vi "Temp Array Gen.2.vi"() -> ()   [LabVIEW 2014]
doc: "Temp Array Gen\n\nCreates an array of temperature given the starting, step, end temperature. This should return an array and the number of temperatures. Takes in consideration inverted limits and steps of zero.\n\nBeverly Abadines\nPHY 350 \nBAP3B"
uses:
  typedefs/temp control params.ctl
panel:
  out "error out":errorcluster
  in  "error in (no error)":errorcluster
  in  "Temperature Control Parameters":T1 {"End Temp" format="%.2f"; "Temp Step" format="%.2f"; "Start Temp" format="%.2f"}
  out "N Temps":i32=6
  out "Temp Array":dbl[](array[numeric])
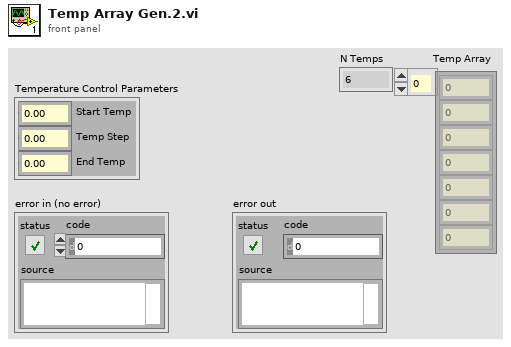
[diagram p1: front panel]
types:
  T1 = typedef "temp control params.ctl" = cluster{"Start Temp":dbl, "Temp Step":dbl, "End Temp":dbl}
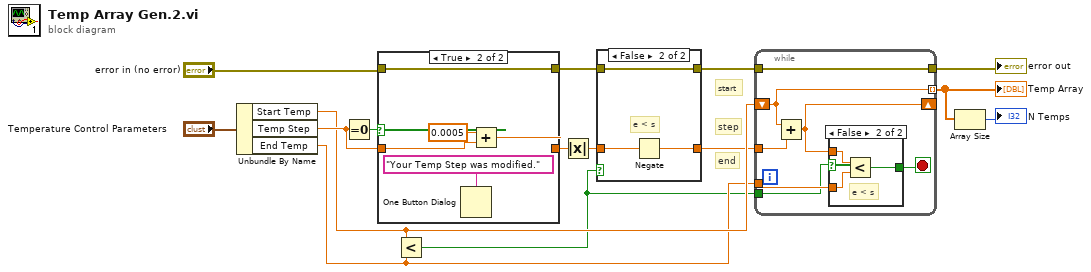
[diagram p0: block diagram]
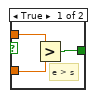
[diagram p4: hidden frame]
diagram:
  # "end"
  # "step"
  # "start"
  n1 = Unbundle By Name("Temperature Control Parameters") -> ("Start Temp"=w8:dbl, "Temp Step"=w11:dbl, "End Temp"=w7:dbl)
  n2 = Equal To 0?(x=w11) -> (x = 0?=w12:bool)
  n3 = case shown="True" w12 {
    tunnel: w11 -> [w17 w22]
    tunnel: [w17 w19] -> w10
    tunnel: "error in (no error)" -> [w16 w18]
    tunnel: [w16 w18] -> w3
    frame False {
    }
    frame True {
      n4 = One Button Dialog(message="Your Temp Step was modified.") -> ()  [unwired: 1 in, 1 out]
      n5 = Add(x=0.0005, y=w22) -> (x+y=w19:dbl)
    }
  }
  n6 = Less?(x=w8, y=w7) -> (x < y?=w5:bool)
  n7 = Absolute Value(x=w10) -> (abs(x)=w9:dbl)
  n8 = case shown="False" w5 {
    tunnel: w9 -> [w24 w27]
    tunnel: [w24 w26] -> w6
    tunnel: w3 -> [w23 w25]
    tunnel: [w23 w25] -> w2
    frame True {
      # "e > s \ngood"
    }
    frame False {
      # "e < s"
      n9 = Negate(x=w27) -> (-x=w26:dbl)
    }
  }
  n10 = while {
    shift-right: [w32] -> _
    shift-left: w8 -> [w34]
    tunnel: [w34] -> w13 mode=indexing
    tunnel: w7 -> [w31]
    tunnel: w6 -> [w33]
    tunnel: w5 -> [w30]
    tunnel: w2 -> [w28]
    tunnel: [w28] -> w1
    stop <- w29 stop-if-true
    n11 = Add(x=w34, y=w33) -> (x+y=w32:dbl)
    n12 = case shown="False" w30 {
      tunnel: w32 -> [w37 w40]
      tunnel: w31 -> [w36 w39]
      tunnel: [w35 w38] -> w29
      frame True {
        # "e > s"
        n13 = Greater?(x=w37, y=w36) -> (0:w35:bool)
      }
      frame False {
        # "e < s"
        n14 = Less?(x=w40, y=w39) -> (x < y?=w38:bool)
      }
    }
  }
  "error out" <- w1
  "Temp Array" <- w13
  n15 = Array Size(array=w13) -> (size(s)=→"N Temps":i32)
